vi "Module Init.vi"(8 "error in (no error)":errorcluster, 11 "Config Alert Module in":refnum<class "Config Monitor Module.lvclass">) -> (0 "error out":errorcluster, 3 "Config Alert Module out":refnum<class "Config Monitor Module.lvclass">)   [LabVIEW 2020, in "VolatusGUI.lvlib" / "Config Monitor Module.lvclass"]
uses:
  Config Monitor Module.lvclass
  C:/dev/lv20CE/relink/lv-volatus/Volatus/Module/Module.lvclass
  Node Config Info.ctl
  Module/Module.lvclass/Module.ctl
  VolatusAPI/VolatusAPI.lvclass/VolatusAPI.ctl
  VolatusConfig/VolatusConfigElement/VolatusConfigElement.lvclass/VolatusConfigElement.ctl
  Config Monitor Module.lvclass/Config Monitor Module.ctl
  VolatusConfig/VolatusConfigElement/Element.vi
  VolatusConfig/Node/Node Config.lvclass
  C:/dev/lv20CE/relink/lv-volatus/VolatusConfig/VolatusConfigElement/VolatusConfigElement.lvclass
  VolatusAPI/VolatusAPI.lvclass
  Module/Module.lvclass
  C:/dev/lv20CE/relink/lv-volatus/Volatus/Config Alert Module/Config Monitor Module.lvclass
  VolatusConfig/Cluster/Cluster Config.lvclass
  VolatusConfig/VolatusConfigElement/VolatusConfigElement.lvclass
  lv-cdm/CDM-Config/Config Element/Config Element.lvclass
  Volatus.lvlib
  C:/dev/lv20CE/relink/lv-volatus/VolatusConfig/Node/Node Config.lvclass
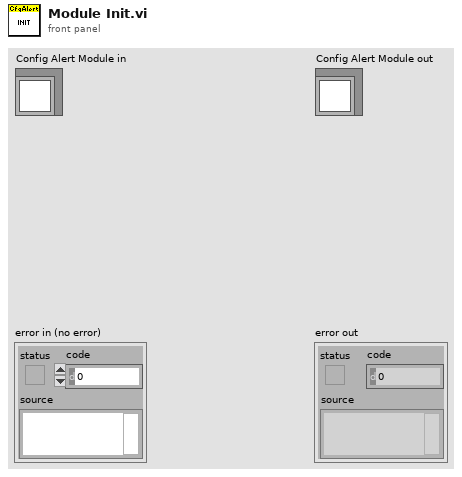
[diagram p1: front panel]
types:
  T1 = typedef "Volatus.lvlib/Node Config Info.ctl" = cluster{"Node":string, "Config Version":string, "Config Hash":string, "Pull":bool, "Push":bool, "Version Color":u32, "Hash Color":u32, "Node Color":u32}
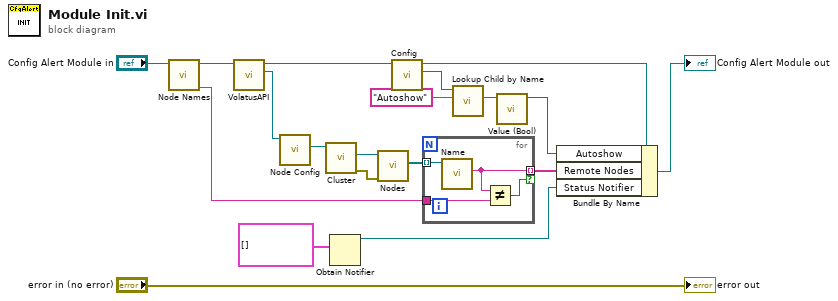
[diagram p0: block diagram]
diagram:
  n1 = call "Node Names.vi"("Module in"="Config Alert Module in") -> ("Node"=w10:string, "Module out"=w14:refnum<class "Config Monitor Module.lvclass">)  [unwired: 6 in, 3 out]
  n2 = call "VolatusAPI.vi"("Module in"=w14) -> ("VolatusAPI"=w16:refnum<class "VolatusAPI.lvclass">, "Module in"=w17:refnum<class "Config Monitor Module.lvclass">)  [unwired: 9 in]
  n3 = call "Node Config.vi"("VolatusAPI in"=w16) -> ("Node Config"=w15:refnum<class "Node Config.lvclass">)  [unwired: 9 in, 1 out]
  n4 = call "Cluster.vi"("Node in"=w15) -> ("error out"=w12:errorcluster, "Cluster"=w13:refnum<class "Cluster Config.lvclass">)  [unwired: 8 in, 1 out]
  n5 = Obtain Notifier(notification data type=T1[] [] ("Array")) -> (notifier out=w1:refnum<notifier>)  [unwired: 3 in, 2 out]
  n6 = call "Nodes.vi"("error in (no error)"=w12, "Cluster in"=w13) -> ("Nodes"=w11:refnum<class "Node Config.lvclass">[])  [unwired: 7 in, 2 out]
  n7 = call "Config.vi"("Module in"=w17) -> ("Config"=w6:refnum<class "VolatusConfigElement.lvclass">, "Module in"=w7:refnum<class "Config Monitor Module.lvclass">)  [unwired: 9 in]
  n8 = for {
    tunnel: w11 -> [w23] mode=indexing
    tunnel: w10 -> [w22]
    tunnel: [w21] -> w8 mode=indexing if=w20
    n9 = call "Name.vi"("VolatusConfigElement in"=w23) -> ("Name"=w21:string)  [unwired: 8 in, 2 out]
    n10 = Not Equal?(x=w21, y=w22) -> (x != y?=w20:bool)
  }
  n11 = call "Lookup Child by Name.vi"("Child Name"="Autoshow", "VolatusConfigElement in"=w6) -> ("Child"=w4:refnum<class "Config Element.lvclass">)  [unwired: 6 in, 3 out]
  n12 = call "Value (Bool).vi"("Config Element in"=w4) -> ("Bool Value"=w3:bool)  [unwired: 9 in, 1 out]
  n13 = Bundle By Name(cluster=w7, "Autoshow"=w3, "Remote Nodes"=w8, "Status Notifier"=w1) -> (→"Config Alert Module out":refnum<class "Config Monitor Module.lvclass">)
  "error out" <- "error in (no error)"
